vi "Write View Data.vi"(8 "error in (no error)":errorcluster, 10 "View Data":string[](array[string]), 11 "List Box View Model In":refnum<class "List Box View Model.lvclass">) -> (0 "error out":errorcluster, 3 "List Box View Model Out":refnum<class "List Box View Model.lvclass">)   [LabVIEW 2020, in "List Box View Model.lvclass"]
uses:
  List Box View Model.lvclass
  List Box View Model.lvclass/List Box View Model.ctl
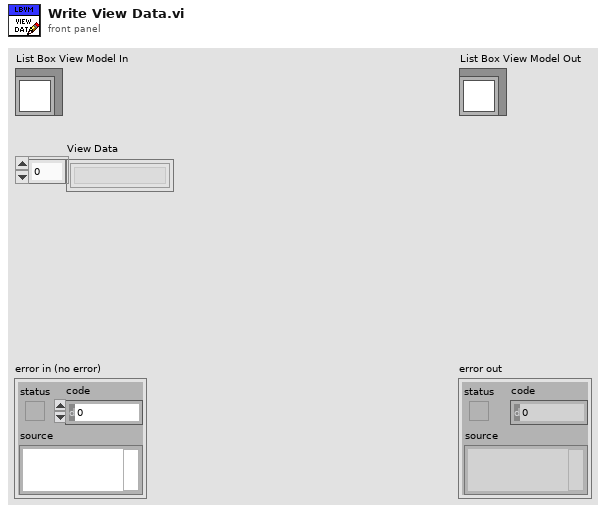
[diagram p1: front panel]
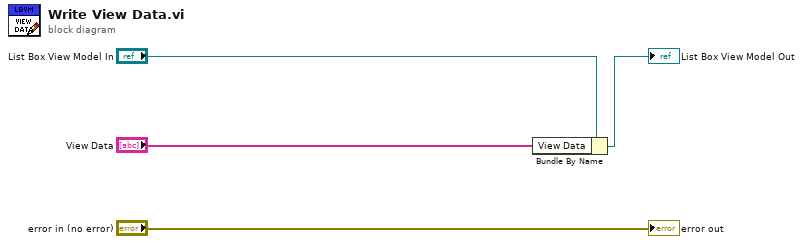
[diagram p0: block diagram]
diagram:
  n1 = Bundle By Name(cluster="List Box View Model In", "View Data"="View Data") -> (→"List Box View Model Out":refnum<class "List Box View Model.lvclass">)
  "error out" <- "error in (no error)"
